vi "Write Command Words.vi"(8 "error in":errorcluster, 10 "command words":T1[](array[typedef]), 11 "Execution Unit in":refnum<class "Execution Unit.lvclass">) -> (0 "error out":errorcluster, 3 "Execution Unit out":refnum<class "Execution Unit.lvclass">)   [LabVIEW 2020, in "Ballard MIL-STD-1553 Engine.lvlib" / "Implementation.lvlib" / "Execution Unit.lvclass"]
uses:
  Execution Unit.lvclass
  Shared/Command Word.ctl
  Execution Unit.lvclass/Execution Unit.ctl
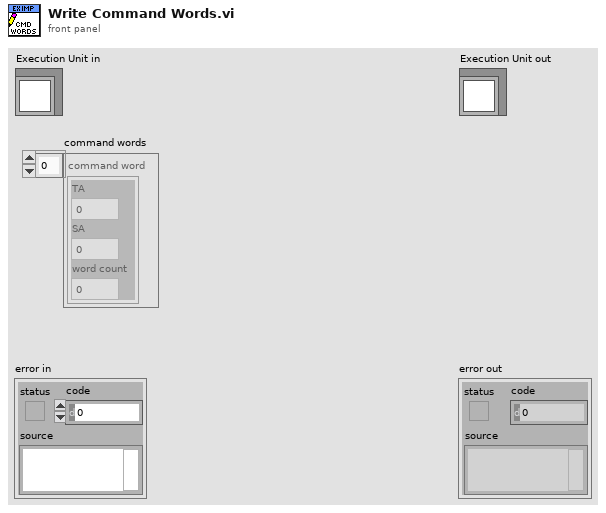
[diagram p1: front panel]
types:
  T1 = typedef "Command Word.ctl" = cluster{"TA":i8, "SA":i8, "word count":i8}
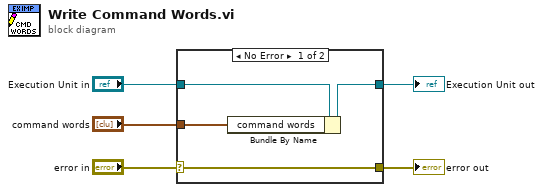
[diagram p0: block diagram]
diagram:
  n1 = case shown="No Error" "error in" {
    selector: "error in" -> [w9 w10]
    tunnel: [w9 w10] -> w4
    tunnel: [w7 w11] -> w2
    tunnel: "Execution Unit in" -> [w8 w11]
    tunnel: "command words" -> [w6 _]
    frame No Error {
      n2 = Bundle By Name(cluster=w8, "command words"=w6) -> (w7:refnum<class "Execution Unit.lvclass">)
    }
    frame Error {
    }
  }
  "error out" <- w4
  "Execution Unit out" <- w2
